vi "215.InitializeMotor (SubVI).vi"() -> ()   [LabVIEW 2020]
panel:
  out "Receive string":string
  out "VISA Out":refnum<visa-resource-name>
  out "Connected":bool
  out "error out":errorcluster
  in  "error in (no error)":errorcluster
  in  "VISA resource name":refnum<visa-resource-name>="COM7"
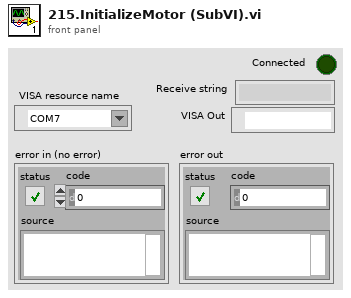
[diagram p1: front panel]
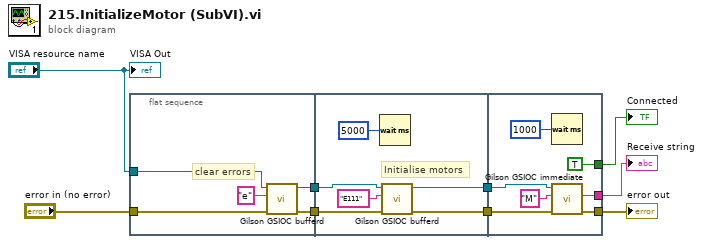
[diagram p0: block diagram]
diagram:
  n1 = flat-sequence {
    tunnel: "error in (no error)" -> [w13]
    tunnel: "VISA resource name" -> [w11]
    tunnel: [w12] -> w8
    tunnel: [w10] -> w9
    tunnel: [w20] -> w7
    tunnel: [w19] -> w6
    tunnel: w9 -> [w16]
    tunnel: w8 -> [w17]
    tunnel: [TRUE] -> w2
    tunnel: w7 -> [w26]
    tunnel: w6 -> [w25]
    tunnel: [w23] -> w3
    tunnel: [w21] -> w1
    frame #0 {
      # "clear errors"
      n2 = call <instrlib>:"Gilson GSIOC bufferd.vi"("error in (no error)"=w13, "Bufferd command"="e", "VISA resource name"=w11) -> ("error out"=w12:errorcluster, "VISA resource name out"=w10:refnum<visa-resource-name>)  [unwired: 6 in, 1 out]
    }
    frame #1 {
      # "Initialise motors"
      n3 = Wait (ms)(milliseconds to wait=u32 5000) -> ()  [unwired: 1 out]
      n4 = call <instrlib>:"Gilson GSIOC bufferd.vi"("error in (no error)"=w17, "Bufferd command"="E111", "VISA resource name"=w16) -> ("error out"=w19:errorcluster, "VISA resource name out"=w20:refnum<visa-resource-name>)  [unwired: 6 in, 1 out]
    }
    frame #2 {
      n5 = Wait (ms)(milliseconds to wait=u32 1000) -> ()  [unwired: 1 out]
      n6 = call <instrlib>:"Gilson GSIOC immediate.vi"("error in (no error)"=w25, "Immediate command"="M", "VISA resource name"=w26) -> ("error out"=w23:errorcluster, "Receive string"=w21:string)  [unwired: 6 in, 1 out]
    }
  }
  "error out" <- w3
  "VISA Out" <- "VISA resource name"
  "Connected" <- w2
  "Receive string" <- w1
